vi "acquire Closed Loop LV.vi"(8 "error in (no error)":errorcluster, 11 "expTime":sgl) -> (0 "error out":errorcluster)   [LabVIEW 2016, in "cameraLibrary.lvlib"]
doc: "Start closed loop camera acquisition, sends corrections to server over TCP.\n\n\n\nvoid CAMERALIBRARYSHARED_EXPORT acquireClosedLoopLV(float expTime);"
uses:
  cameraLibrary.lvlib
  cameraLibrary.dll
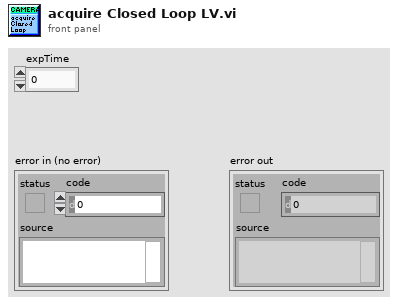
[diagram p1: front panel]
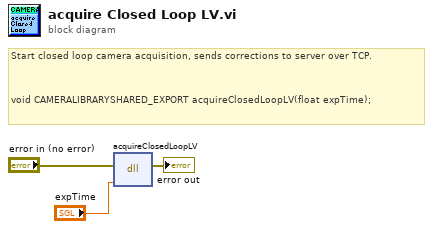
[diagram p0: block diagram]
diagram:
  # "Start closed loop camera acquisition, sends corrections to server over TCP.\n\n\n\nvoid CAMERALIBRARYSHARED_EXPORT acquireClosedLoopLV(float expTime);"
  n1 = dll-call lib="C:/Users/TMM/repos/EXPRES/FEM/FTT/support/Camera Library/cameraLibrary.*" fn="acquireClosedLoopLV"(error in="error in (no error)", "expTime"="expTime") -> (error out=→"error out":errorcluster)  [unwired: 4 in, 1 out]
